vi "ReceiveWaveform.vi"(8 "error in (no error)":errorcluster, 10 "Waveform":waveform(dbl), 11 "TransferData in":refnum<class "TransferData.lvclass">) -> (0 "error out":errorcluster, 3 "TransferData out":refnum<class "TransferData.lvclass">)   [LabVIEW 2020, in "SimDaq.lvlib" / "TransferData.lvclass"]
uses:
  TransferData.lvclass
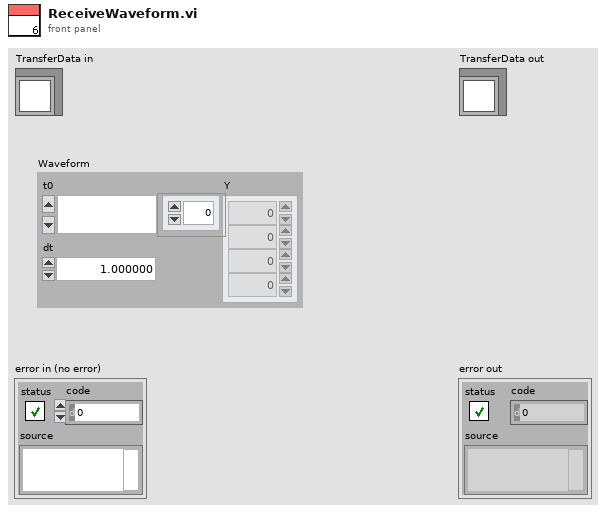
[diagram p1: front panel]
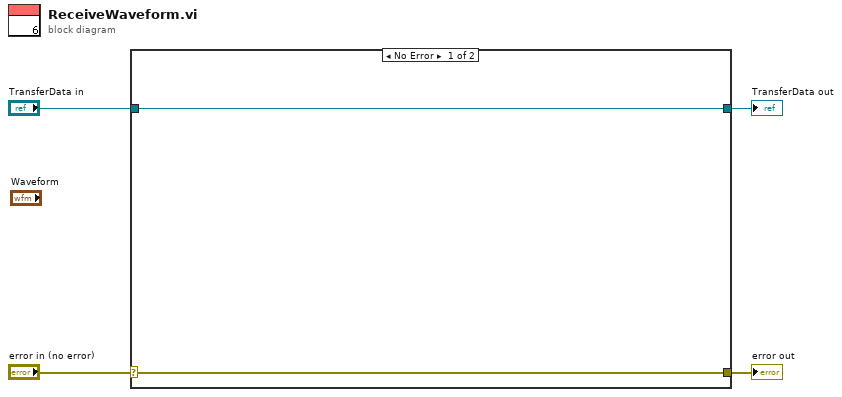
[diagram p0: block diagram]
diagram:
  n1 = case shown="No Error" "error in (no error)" {
    selector: "error in (no error)" -> [w5 w8]
    tunnel: [w5 w8] -> w3
    tunnel: [w6 w7] -> w1
    tunnel: "TransferData in" -> [w6 w7]
    frame No Error {
    }
    frame Error {
    }
  }
  "error out" <- w3
  "TransferData out" <- w1
